vi "RVC Rotate Animation.vi"() -> ()   [LabVIEW 2013]
uses:
  <vilib>/Analysis/baseanly.llb/Real A x B.vi
  <vilib>/Analysis/baseanly.llb/Dot Product.vi
  <vilib>/Analysis/baseanly.llb/Real Dot Product.vi
  <vilib>/Analysis/baseanly.llb/Outer Product.vi
  <vilib>/Analysis/baseanly.llb/Real Outer Product.vi
  <vilib>/robotics/Kinematics/Create Lie Group Matrix.vi
  <vilib>/robotics/Kinematics/Rotation Matrix to Angle Vector.vi
  <vilib>/Analysis/Matrix/Numeric/Multiply/Multiply.vi
  <vilib>/Analysis/Matrix/Numeric/Multiply/Multiply - RM,R.vi
  <vilib>/Analysis/Matrix/Numeric/Multiply/Multiply - R,RM.vi
  <vilib>/Analysis/Matrix/Numeric/Add/Add.vi
  <vilib>/Analysis/Matrix/Numeric/Add/Add - RM,RM.vi
  <vilib>/robotics/Kinematics/NI_Kinematics.lvlib
  <vilib>/Analysis/NI_AALBase.lvlib
panel:
  out "3D Picture 2":refnum<vi>(3d-picture)
  out "rot X * rot Y":picture
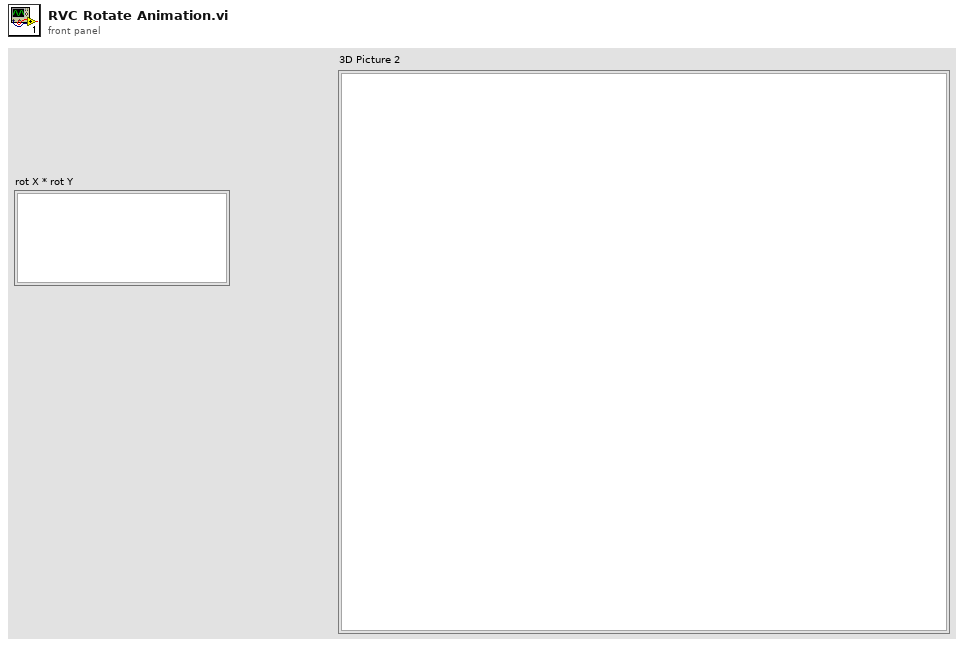
[diagram p1: front panel]
types:
  T1 = typedef "NI_Matrix.lvlib/RealMatrix.ctl" = dbl[][]
  T2 = typedef "NI_Kinematics.lvlib/Quaternion.ctl" = dbl[]
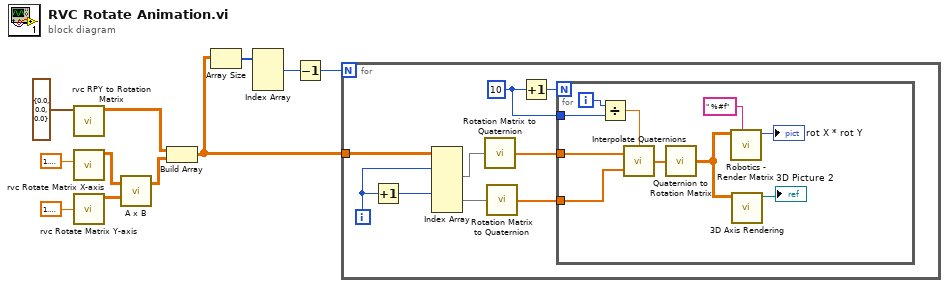
[diagram p0: block diagram]
diagram:
  n1 = call "rvc RPY to Rotation Matrix.vi"("angles"=cluster{"roll":dbl, "pitch":dbl, "yaw":dbl} {"roll"=0.0, "pitch"=0.0, "yaw"=0.0}) -> ("rotation matrix"=w8:T1)  [unwired: 10 in]
  n2 = call "rvc Rotate Matrix X-axis.vi"("angle"=1.5707963267948966) -> ("rotation matrix"=w3:T1)  [unwired: 10 in]
  n3 = call "rvc Rotate Matrix Y-axis.vi"("angle"=1.5707963267948966) -> ("rotation matrix"=w2:T1)  [unwired: 10 in]
  n4 = call-poly <vilib>:"A x B.vi"("B"=w2, "A"=w3) -> ("A x B"=w1:T1)  [unwired: 1 out]
  n5 = Build Array(w8, w1) -> (w7:dbl[][][])
  n6 = Array Size(array=w7) -> (size(s)=w6:i32[])
  n7 = Index Array(array=w6) -> (element #1=w5:i32)  [unwired: 3 in, 2 out]
  n8 = Decrement(x=w5) -> (x-1=w4:i32)
  n9 = for {
    N: w4 -> [_]
    tunnel: w7 -> [w19]
    i -> [w16]
    w12 = 10
    n10 = Increment(x=w16) -> (x+1=w17:i32)
    n11 = Index Array(array=w19, index (dim 0) #1=w16, index (dim 0) #2=w17) -> (element #1=w18:dbl[][], element #2=w15:dbl[][])  [unwired: 4 in]
    n12 = call <vilib>:"Rotation Matrix to Quaternion.vi"("rotation matrix"=w18) -> ("quaternion"=w20:T2)
    n13 = call <vilib>:"Rotation Matrix to Quaternion.vi"("rotation matrix"=w15) -> ("quaternion"=w14:T2)
    n14 = Increment(x=w12) -> (x+1=w13:i32)
    n15 = for {
      N: w13 -> [_]
      tunnel: w20 -> [w22]
      tunnel: w14 -> [w21]
      tunnel: w12 -> [w23]
      i -> [w24]
      n16 = Divide(x=w24, y=w23) -> (x/y=w27:dbl)
      n17 = call <vilib>:"Interpolate Quaternions.vi"("ratio"=w27, "quaternion 2"=w21, "quaternion 1"=w22) -> ("interpolated quaternion"=w26:T2)
      n18 = call <vilib>:"Quaternion to Rotation Matrix.vi"("quaternion"=w26) -> ("rotation matrix"=w25:T1)
      n19 = call "Robotics - Render Matrix.vi"("format string"=" %#f", "A"=w25) -> ("picture out"=→"rot X * rot Y":picture)  [unwired: 9 in]
      n20 = call "3D Axis Rendering.vi"("rotation matrix"=w25) -> ("SceneNode out"=→"3D Picture 2":refnum<vi>)  [unwired: 9 in, 1 out]
    }
  }
